vi "Load Previous Command.vi"(0 "Number of LBCBs":T1) -> ()   [LabVIEW 2009]
uses:
  lib/Data Access Objects/Application/Number Of LBCBs.ctl
  lib/Apps/App Parameters Actions.ctl
  lib/Data Access Objects/Metadata/DAO Actions.ctl
  lib/Data Access Objects/Metadata/LBCB Number.ctl
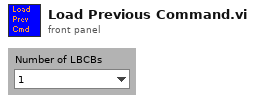
[diagram p1: front panel]
types:
  T1 = typedef "Number Of LBCBs.ctl" = enum16{"1", "2"}
  T2 = typedef "App Parameters Actions.ctl" = enum16{"Init", "Get", "Set"}
  T3 = typedef "App Parameters.ctl" = cluster{"Monitor Loop":T4, "Ramp Time":T4, "Log Loop":T4, "TCP to DAQ":T4, "Logging Directory":path, "Log File Size (MBytes)":i64, "Volt Logging Loop":T4}
  T4 = typedef "Timing Parameters.ctl" = cluster{"Interval":dbl, "Rate ":dbl}
  T5 = typedef "LBCB Number.ctl" = enum16{"LBCB1", "LBCB2"}
  T6 = enum16{"open", "replace", "create", "open or create", "replace or create", "replace or create with confirmation"}
  T7 = typedef "DAO Actions.ctl" = enum16{"Init", "Get", "Set"}
  T8 = typedef "Actuator Point.ctl" = cluster{"X1":dbl, "X2":dbl, "Y1":dbl, "Z1":dbl, "Z2":dbl, "Z3":dbl}
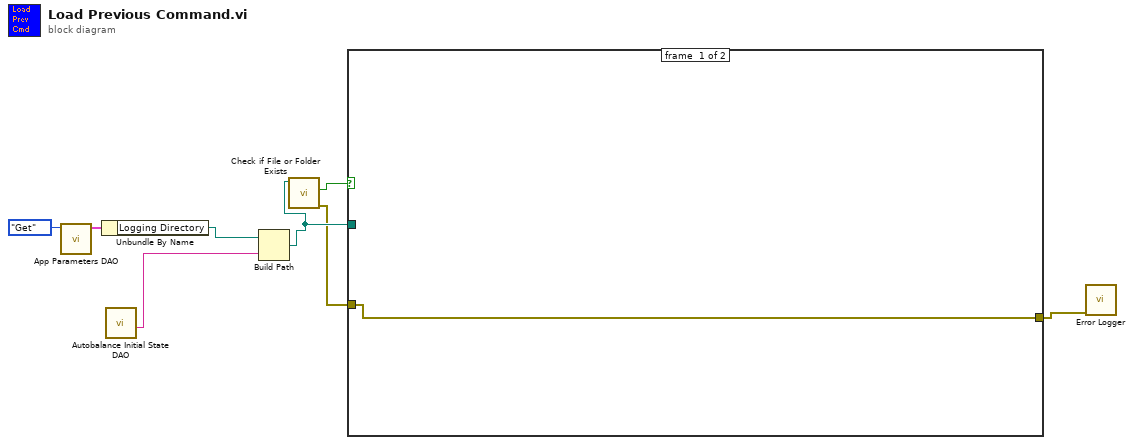
[diagram p0: block diagram]
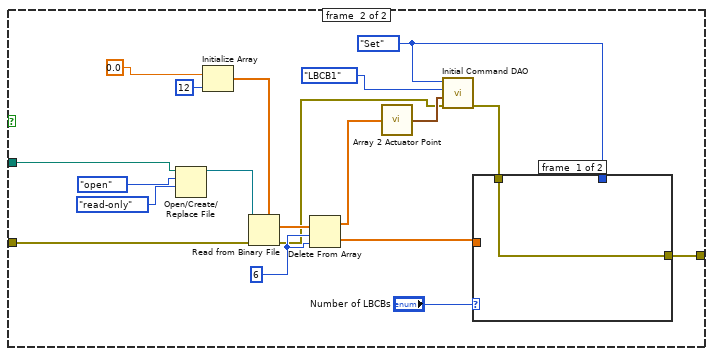
[diagram p2: hidden frame]
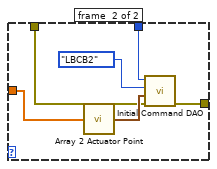
[diagram p3: hidden frame]
diagram:
  n1 = call "App Parameters DAO.vi"("Actions"=App_Parameters_Actions."Get" ("App Parameter Actions")) -> ("Application Timing and Logging Out"=w6:T3)  [unwired: 3 in, 7 out]
  n2 = Unbundle By Name(w6) -> ("Logging Directory"=w7:path)
  n3 = call "Autobalance Initial State DAO.vi"() -> ("autobalance\nfile"=w8:string)  [unwired: 2 in, 9 out]
  n4 = Build Path(base path=w7, name or relative path=w8) -> (appended path=w3:path)
  n5 = call <vilib>:"Check if File or Folder Exists.vi"("path"=w3) -> ("error out"=w1:errorcluster, "file or folder exists?"=w4:bool)  [unwired: 1 in, 8 out]
  n6 = case shown="True" w4 {
    tunnel: w3 -> [_ w19]
    tunnel: [w9 w11] -> w2
    tunnel: w1 -> [w9 w10]
    frame #0 {
    }
    frame #1 {
      w14 = DAO_Actions."Set" ("DAO Actions")
      w21 = 6 ("length")
      n7 = Open/Create/Replace File(file path (use dialog)=w19, operation (0:open)=T6."open", access (0:read/write)=enum16{"read/write", "read-only", "write-only"}."read-only") -> (refnum out=w28:refnum<file>)  [unwired: 1 in, 4 out]
      n8 = Initialize Array(0.0, 12 ("dimension size")) -> (w23:dbl[])
      n9 = Read from Binary File(5:w23, 8:w10, 11:w28) -> (0:w13:errorcluster, 2:w22:dbl[])  [unwired: 5 out]
      n10 = Delete From Array(array=w22, length=w21, index=w21) -> (deleted portion=w20:dbl[], array with subset deleted=w16:dbl[])
      n11 = call "Array 2 Actuator Point.vi"("Array"=w16) -> ("Actuator Point"=w15:T8)
      n12 = call "Initial Command DAO.vi"("error in (no error)"=w13, "Command In"=w15, "LBCB Number"=LBCB_Number."LBCB1" ("Selected LBCB"), "DAO Actions"=w14) -> ("error out"=w12:errorcluster)  [unwired: 7 out]
      n13 = case shown="\"1\"" "Number of LBCBs" {
        tunnel: w20 -> [_ w35]
        tunnel: w14 -> [_ w33]
        tunnel: w12 -> [w29 w31]
        tunnel: [w29 w30] -> w11
        frame #0 {
        }
        frame #1 {
          n14 = call "Array 2 Actuator Point.vi"("Array"=w35) -> ("Actuator Point"=w34:T8)
          n15 = call "Initial Command DAO.vi"("error in (no error)"=w31, "Command In"=w34, "LBCB Number"=LBCB_Number."LBCB2" ("Selected LBCB"), "DAO Actions"=w33) -> ("error out"=w30:errorcluster)  [unwired: 7 out]
        }
      }
    }
  }
  n16 = call "Error Logger.vi"("error in (no error)"=w2) -> ()  [unwired: 1 in, 10 out]
